vi "NI_FPGA_PPG.load.vi"(0 "i ref in":refnum<vi>, 2 "cmd_data_string":string, 3 "ms timeout (10000)":i32=10000, 5 "error in (no error)":errorcluster) -> (14 "i ref out":refnum<vi>, 17 "timed out":bool, 19 "error out":errorcluster)   [LabVIEW 2014, in "NI_FPGA_PPG.lvlib"]
doc: "Loads complete command sequence (see command syntax) to the FPGA target.\n\nLicense Agreement for this software:\n\nCopyright (C) 2009\nFalk Ziegler\nInstitut für Physik\nErnst-Moritz-Arndt Universität\nFelix-Hausdorff-Str. 6\n17487 Greifswald\n\nContact: Falk Ziegler, ziegler@physik.uni-greifswald.de\n\nThis program is free software: you can redistribute it and/or modify it under the terms of the GNU General Public License as published by the Free Software Foundation, either version 3 of the License, or (at your option) any later version.\n\nThis program is distributed in the hope that it will be useful, but WITHOUT ANY WARRANTY; without even the implied warranty of MERCHANTABILITY or FITNESS FOR A PARTICULAR PURPOSE. See the GNU General Public License for more details.\n\nYou should have received a copy of the GNU General Public License along with this program. If not, see <http://www.gnu.org/licenses/>.\n\nFor all questions and ideas contact: ziegler@physik.uni-greifswald.de or d.beck@gsi.de\nLast update: 01-Sep-2009"
uses:
  NI_FPGA_PPG.lvlib
  CSCore/CSApplicationBaseClasses/DeviceBase/DeviceBase.lvlib
  CSinstr.lib/NI-FPGA-PPG/host/instrumentDriver/NI-FPGA-PPG_Driver.lvlib
  CSCore/CSSystem/CoreLib/CoreLib.lvlib
  CSlibraries/UtilityLib/UtilityLib.lvlib
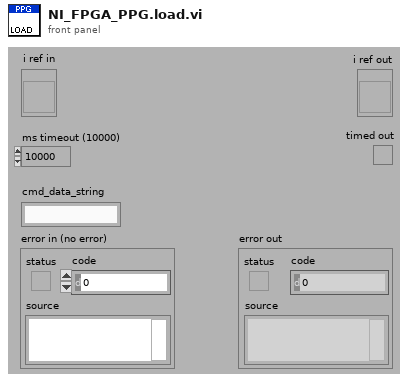
[diagram p1: front panel]
types:
  T1 = typedef "NI_FPGA_PPG.lvlib/NI_FPGA_PPG.i attribute.ctl" = cluster{"dim_service_id":cluster{"dim_actual_device_status":i32, "dim_event_data":i32, "dim_cmd_data":i32, "dim_cmd_data _description":i32, "dim_channel_description":i32}, "VISA":refnum<visa-resource-name>, "actual_device_status":i32, "event_data_id":i32, "pdc_enabled":bool, "pdc_timestamp":u32, "cmd_data_string":string, "cmd_data_size":i32, "cmd_data_description_string":string, "cmd_data_description_size":i32, "channel_description_string":string, "channel_description_size":i32}
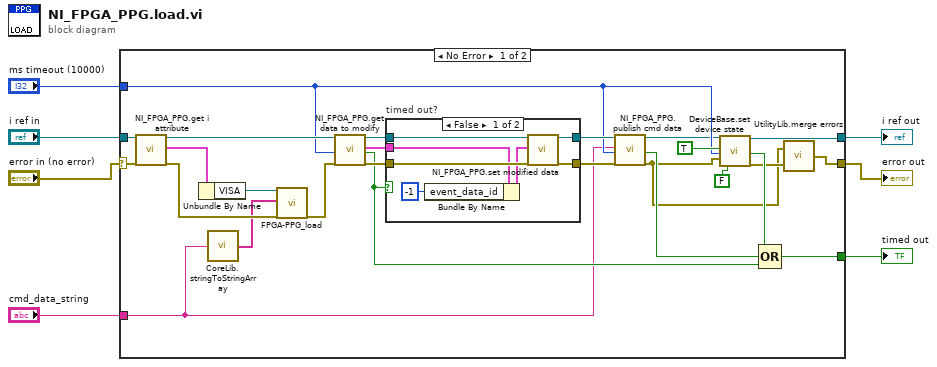
[diagram p0: block diagram]
diagram:
  n1 = case shown="No Error" "error in (no error)" {
    selector: "error in (no error)" -> [w32 w43]
    tunnel: "i ref in" -> [w33 w44]
    tunnel: [w26 w44] -> w5
    tunnel: [w8 w43] -> w4
    tunnel: "ms timeout (10000)" -> [w15 _]
    tunnel: "cmd_data_string" -> [w11 _]
    tunnel: [w19 _] -> w1
    frame No Error {
      n2 = call "NI_FPGA_PPG.get i attribute.vi"("i ref in"=w33, "error in (no error)"=w32) -> ("i ref out"=w25:refnum<vi>, "i attribute"=w31:T1, "error out"=w29:errorcluster)  [unwired: 15 in]
      n3 = Unbundle By Name(w31) -> ("VISA"=w30:refnum<visa-resource-name>)
      n4 = call "CoreLib.stringToStringArray.vi"("String"=w11) -> ("Array"=w12:string[])
      n5 = call "FPGA-PPG_load.vi"("resource_in"=w30, "command_lines"=w12, "error in (no error)"=w29) -> ("error out"=w13:errorcluster)  [unwired: 15 in, 1 out]
      n6 = call "NI_FPGA_PPG.get data to modify.vi"("i ref in"=w25, "ms timeout (10000)"=w15, "error in (no error)"=w13) -> ("i ref out"=w24:refnum<vi>, "i attribute"=w22:T1, "timed out"=w20:bool, "error out"=w23:errorcluster)  [unwired: 13 in]
      n7 = case "timed out?" shown="False" w20 {
        tunnel: w24 -> [w40 w42]
        tunnel: w23 -> [w39 w41]
        tunnel: w22 -> [w38 _]
        tunnel: [w35 w42] -> w18
        tunnel: [w34 w41] -> w17
        frame False {
          n8 = Bundle By Name(cluster=w38, "event_data_id"=-1) -> (w37:T1)
          n9 = call "NI_FPGA_PPG.set modified data.vi"("i ref in"=w40, "i attribute"=w37, "error in (no error)"=w39) -> ("i ref out"=w35:refnum<vi>, "error out"=w34:errorcluster)  [unwired: 15 in]
        }
        frame True {
        }
      }
      n10 = call "NI_FPGA_PPG.publish cmd data.vi"("i ref in"=w18, "cmd_data_string"=w11, "ms timeout (10000)"=w15, "error in (no error)"=w17) -> ("i ref out"=w14:refnum<vi>, "timed out"=w16:bool, "error out"=w9:errorcluster)  [unwired: 13 in]
      n11 = call "DeviceBase.set device state.vi"("i ref in"=w14, "implicit"=TRUE, "ms timeout (10000)"=w15, "device error"=w9, "mayResetError (FALSE)"=FALSE) -> ("i ref out"=w26:refnum<vi>, "timed out"=w21:bool, "error out"=w10:errorcluster)  [unwired: 12 in]
      n12 = Compound Arithmetic op=OR(w21, w16, w20) -> (w19:bool)
      n13 = call "UtilityLib.merge errors.vi"("error2 (no error)"=w10, "error1 (no error)"=w9) -> ("error out"=w8:errorcluster)
    }
    frame Error {
    }
  }
  "error out" <- w4
  "i ref out" <- w5
  "timed out" <- w1
